vi "LVObject to JSON - Recursion - Returns No Error.vi"() -> ()   [LabVIEW 2017, in "JSON Serializable Serializer Tests.lvlib"]
uses:
  JSON Serializable Serializer Tests.lvlib
  JSON Serializable Serializer/JSON Serializable Serializer.lvclass
  <vilib>/addons/_JKI Toolkits/Caraya/classes/Assert/Assert Not Error.vi
  <vilib>/addons/_JKI Toolkits/Caraya/classes/Test/Test.lvclass
  <vilib>/addons/_JKI Toolkits/Caraya/classes/Assert/Assert.lvclass
  Recursive JSON Serializable/Recursive JSON Serializable.lvclass
panel:
  out "<JSON>Object":string
  out "error out":errorcluster
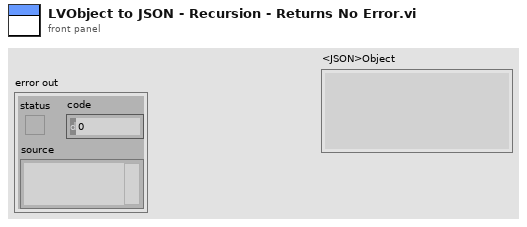
[diagram p1: front panel]
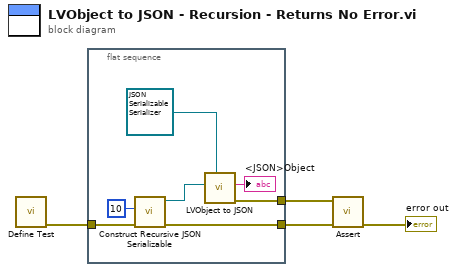
[diagram p0: block diagram]
diagram:
  n1 = call <vilib>:"Define Test.vi"() -> ("error out"=w3:errorcluster)  [unwired: 11 in]
  n2 = flat-sequence {
    tunnel: [w11] -> w1
    tunnel: [w8] -> w4
    tunnel: w3 -> [w10]
    frame #0 {
      n3 = call "Construct Recursive JSON Serializable.vi"("error in (no error)"=w10, "Recursion Level"=u8 10) -> ("error out"=w8:errorcluster, "Recursive JSON Serializable"=w7:refnum<class "Recursive JSON Serializable.lvclass">)  [unwired: 8 in]
      n4 = call-dynamic "LVObject to JSON.vi"("JSON Serializable Serializer in"=refnum<class "JSON Serializable Serializer.lvclass"> refnum ("JSON Serializer.lvclass"), "Object"=w7) -> ("error out"=w11:errorcluster, "<JSON>Object"=→"<JSON>Object":string)  [unwired: 8 in]
    }
  }
  n5 = call-poly <vilib>:"Assert.vi"("error in (no error)"=w4, "Not Error?"=w1) -> ("error out"=→"error out":errorcluster)  [unwired: 9 in]
